vi "Set Image Flip.vi"(8 "error in (no error)":errorcluster, 10 "iVFlip":i32, 11 "iHFlip":i32) -> (0 "error out":errorcluster, 3 "function return":u32)   [LabVIEW 2014, in "atmcd32d.lvlib"]
doc: "unsigned int WINAPI SetImageFlip(int iHFlip, int iVFlip);"
uses:
  atmcd32d.lvlib
  atmcd32d.dll
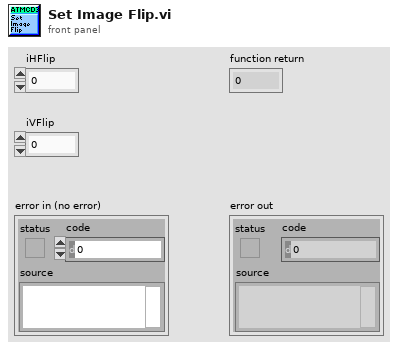
[diagram p1: front panel]
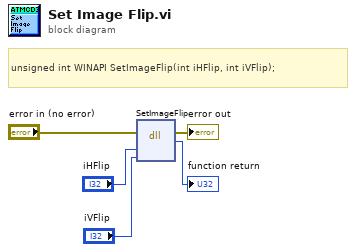
[diagram p0: block diagram]
diagram:
  # "unsigned int WINAPI SetImageFlip(int iHFlip, int iVFlip);"
  n1 = dll-call lib="C:/Users/Bakir/Documents/Lambda2-Testing/lib/Andorlib/atmcd32d.*" fn="SetImageFlip"(error in="error in (no error)", "iHFlip"="iHFlip", "iVFlip"="iVFlip") -> (error out=→"error out":errorcluster, →"function return":u32)  [unwired: 4 in, 1 out]
